vi "Initialise.vi"(2 "error in (no error)":errorcluster, 3 "Facing":dbl, 4 "Y":dbl, 5 "X":dbl) -> (0 "error out":errorcluster, 1 "SonarSensor.lvclass":refnum<class "SonarSensor.lvclass">)   [LabVIEW 2015, in "SonarSensor.lvclass"]
uses:
  SonarSensor.lvclass
  Sensor.lvclass
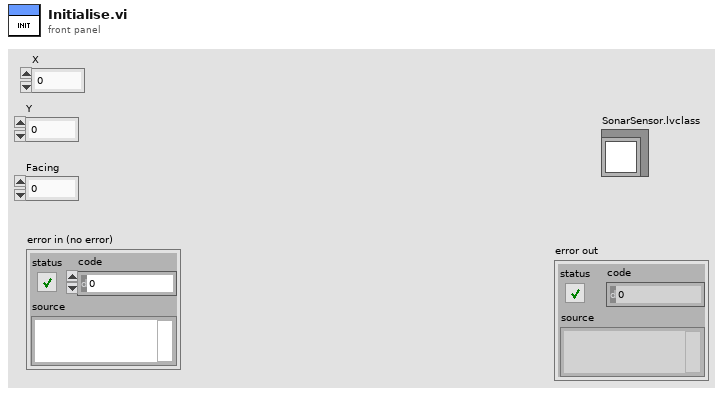
[diagram p1: front panel]
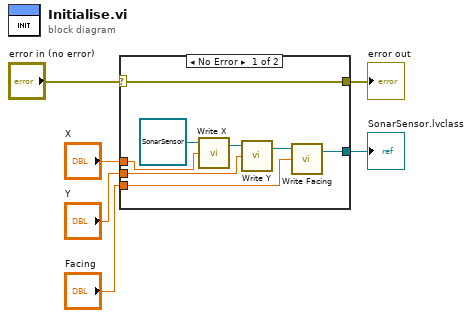
[diagram p0: block diagram]
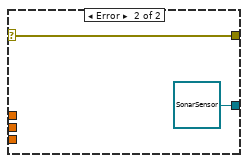
[diagram p2: hidden frame]
diagram:
  n1 = case shown="No Error" "error in (no error)" {
    selector: "error in (no error)" -> [w7 w15]
    tunnel: "X" -> [w13 _]
    tunnel: "Y" -> [w11 _]
    tunnel: "Facing" -> [w9 _]
    tunnel: [w8 refnum<class "SonarSensor.lvclass"> refnum ("SonarSensor.lvclass")] -> w2
    tunnel: [w7 w15] -> w1
    frame No Error {
      n2 = call "Write X.vi"("X"=w13, "Sensor In"=refnum<class "SonarSensor.lvclass"> refnum ("SonarSensor.lvclass")) -> ("Sensor Out"=w12:refnum<class "SonarSensor.lvclass">)  [unwired: 1 in, 1 out]
      n3 = call "Write Y.vi"("Y"=w11, "Sensor In"=w12) -> ("Sensor Out"=w10:refnum<class "SonarSensor.lvclass">)  [unwired: 1 in, 1 out]
      n4 = call "Write Facing.vi"("Facing"=w9, "Sensor.lvclass"=w10) -> ("Sensor.lvclass"=w8:refnum<class "SonarSensor.lvclass">)  [unwired: 1 in, 1 out]
    }
    frame Error {
    }
  }
  "error out" <- w1
  "SonarSensor.lvclass" <- w2
